vi "Creator Queue.vi"(9 "Priority?":bool, 10 "Msg Strategy":refnum<class "Msg Strategy.lvclass">, 11 "Hello World Queue in":refnum<class "Hello World Queue.lvclass">) -> (3 "Hello World Queue out":refnum<class "Hello World Queue.lvclass">)   [LabVIEW 2021, in "Hello World Queue.lvlib" / "Hello World Queue.lvclass"]
uses:
  Hello World Queue.lvclass
  jettl/Msg Strategy/Msg Strategy.lvclass
  Hello World Queue.lvclass/Hello World Queue.ctl
  jettl/Queue jettl/Queue jettl.lvclass
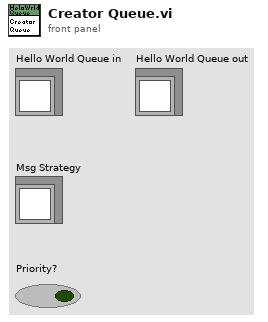
[diagram p1: front panel]
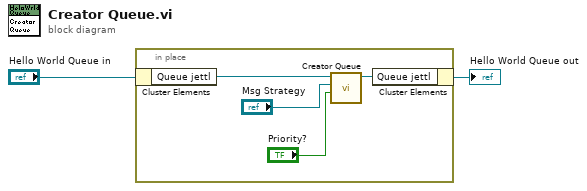
[diagram p0: block diagram]
diagram:
  n1 = in-place {
    n2 = in-place-cluster #1("Hello World Queue in") -> ("Queue jettl"=w6:refnum<class "Queue jettl.lvclass">)
    n3 = call-dynamic "Creator Queue.vi"("Priority?"="Priority?", "Msg Strategy"="Msg Strategy", "Queue jettl in"=w6) -> ("Queue jettl out"=w5:refnum<class "Queue jettl.lvclass">)  [unwired: 8 in]
    n4 = in-place-cluster #1("Queue jettl"=w5) -> (→"Hello World Queue out":refnum<class "Hello World Queue.lvclass">)
  }
